vi "Write tsignalonsensor elements u bazu_Core.vi"() -> ()   [LabVIEW 2011]
uses:
  <vilib>/addons/database/Connection.llb/DB Tools Open Connec (String).vi
  <vilib>/addons/database/NI_Database_API.lvlib
panel:
  out "error out":errorcluster
  out "Array":i32[][](array[numeric])
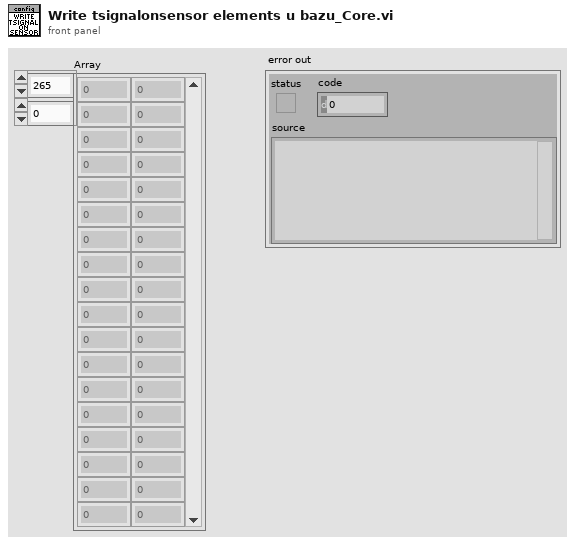
[diagram p1: front panel]
types:
  T1 = typedef "NI_Database_API.lvlib/Conn ObjectReference.ctl" = refnum<k1>
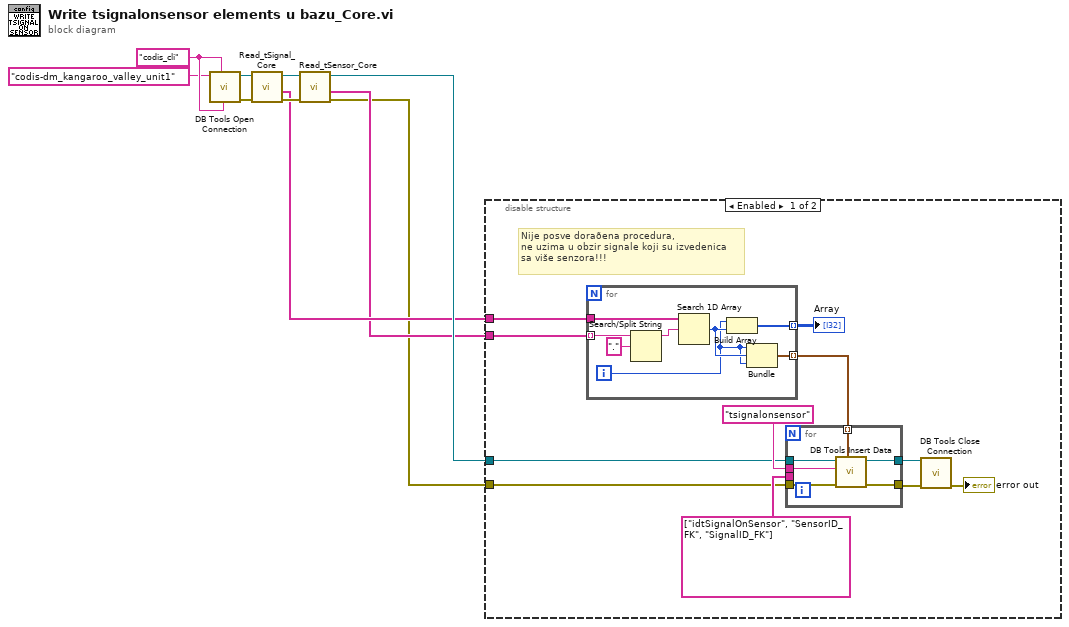
[diagram p0: block diagram]
diagram:
  w10 = "codis_cli" ("userID")
  n1 = call-poly <vilib>:"DB Tools Open Connection.vi"("password"=w10, "userID"=w10, "connection information"="codis-dm_kangaroo_valley_unit1" ("userID")) -> ("error out"=w7:errorcluster, "connection reference"=w9:T1)  [unwired: 5 in]
  n2 = call "Read_tSignal_Core.vi"("error in (no error)"=w7, "connection reference IN"=w9) -> ("error out"=w6:errorcluster, "SignalLabel OUT"=w4:string[], "connection reference OUT"=w8:T1)  [unwired: 5 in, 2 out]
  n3 = call "Read_tSensor_Core.vi"("error in (no error)"=w6, "connection reference IN"=w8) -> ("error out"=w2:errorcluster, "SensorLabel OUT"=w3:string[], "connection reference out"=w5:T1)  [unwired: 5 in, 2 out]
  n4 = disable-structure shown="Enabled" {
    disable-tunnel: w3 -> [w21 _]
    disable-tunnel: w4 -> [w20 _]
    disable-tunnel: w5 -> [w12 _]
    disable-tunnel: w2 -> [w11 _]
    frame Enabled {
      # "Nije posve doraðena procedura,\nne uzima u obzir signale koji su izvedenica\nsa više senzora!!!"
      n5 = for {
        tunnel: w21 -> [w35] mode=indexing
        tunnel: w20 -> [w32]
        tunnel: [w31] -> w19 mode=indexing
        tunnel: [w30] -> w13 mode=indexing
        i -> [w28]
        n6 = Search/Split String(string=w35, search string/char (-)=".") -> (substring before match=w33:string)  [unwired: 1 in, 2 out]
        n7 = Search 1D Array(1D array=w32, element=w33) -> (index of element=w29:i32)  [unwired: 1 in]
        n8 = Build Array(w28, w29) -> (w31:i32[])
        n9 = Bundle(w28, "index of element"=w29, w28) -> (w30:cluster{i32, "index of element":i32, i32})  [unwired: 1 in]
      }
      "Array" <- w19
      n10 = for {
        tunnel: w12 -> [w27]
        tunnel: w11 -> [w26]
        tunnel: "tsignalonsensor" ("table") -> [w25]
        tunnel: w13 -> [w24] mode=indexing
        tunnel: [w23] -> w14
        tunnel: [w22] -> w15
        tunnel: string[] ["idtSignalOnSensor", "SensorID_FK", "SignalID_FK"] ("columns") -> [_]
        n11 = call <vilib>:"DB Tools Insert Data.vi"("data"=w24, "error in (no error)"=w26, "table"=w25, "connection reference"=w27) -> ("error out"=w23:errorcluster, "connection reference out"=w22:T1)  [unwired: 6 in]
      }
      n12 = call <vilib>:"DB Tools Close Connection.vi"("error in (no error)"=w14, "connection reference"=w15) -> ("error out"=→"error out":errorcluster)  [unwired: 5 in]
    }
    frame Disabled {
    }
  }
